vi "Write AI_Config.vi"(8 "error in (no error)":errorcluster, 10 "AI_Config":T1={"MaxValue"=1.0, "MinValue"=0.0, "InputTerminalConfiguration"=-1} {"InputTerminalConfiguration" items=["default"=-1, "RSE"=10083, "NRSE"=10078, "Differential"=10106, "Pseudodifferential"=12529]}, 11 "AI_Task in":refnum<class "AI_Task.lvclass">) -> (0 "error out":errorcluster, 3 "AI_Task out":refnum<class "AI_Task.lvclass">)   [LabVIEW 2025, in "AI_Task.lvlib" / "AI_Task.lvclass"]
uses:
  AI_Task.lvclass
  AI_Task.lvclass/AI_Task.ctl
  DAQ_Module/DAQ_Module/DAQ_Module/DAQ_AI_Task_Config.ctl
  DAQ_Module/DAQ_Module/DAQ_Module/DAQ_Module.lvclass
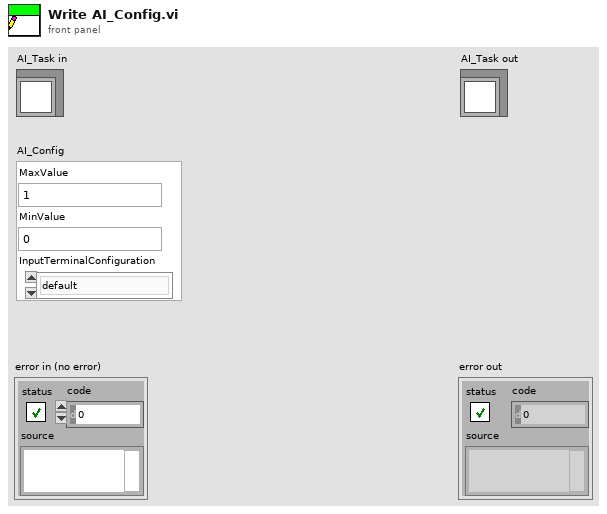
[diagram p1: front panel]
types:
  T1 = typedef "DAQ_Module.lvlib/DAQ_Module.lvclass/DAQ_AI_Task_Config.ctl" = cluster{"MaxValue":dbl, "MinValue":dbl, "InputTerminalConfiguration":i32}
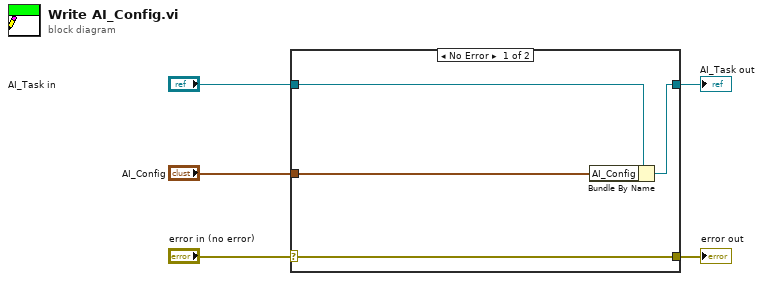
[diagram p0: block diagram]
diagram:
  n1 = case shown="No Error" "error in (no error)" {
    selector: "error in (no error)" -> [w9 w10]
    tunnel: [w9 w10] -> w4
    tunnel: [w7 w11] -> w2
    tunnel: "AI_Task in" -> [w8 w11]
    tunnel: "AI_Config" -> [w6 _]
    frame No Error {
      n2 = Bundle By Name(cluster=w8, "AI_Config"=w6) -> (w7:refnum<class "AI_Task.lvclass">)
    }
    frame Error {
    }
  }
  "error out" <- w4
  "AI_Task out" <- w2
